vi "OFDM-A2信道估计.vi"(1 "信道2导频输入":cdb[](array[numeric])) -> (0 "输出":cdb[](array[numeric]))   [LabVIEW 2018]
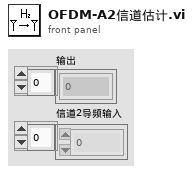
[diagram p1: front panel]
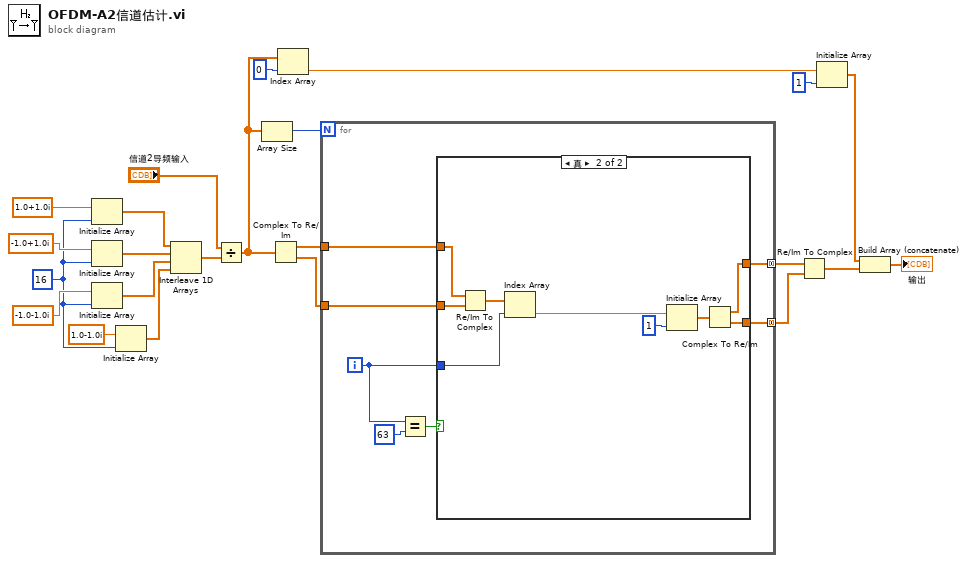
[diagram p0: block diagram]
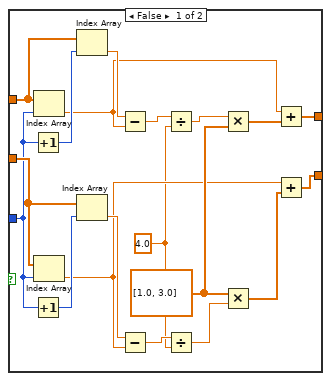
[diagram p2: hidden frame]
diagram:
  w2 = 16
  n1 = Initialize Array(cdb 1.0+1.0i, w2) -> (w9:cdb[])
  n2 = Initialize Array(cdb -1.0+1.0i, w2) -> (w6:cdb[])
  n3 = Initialize Array(cdb -1.0-1.0i, w2) -> (w7:cdb[])
  n4 = Initialize Array(cdb 1.0-1.0i, w2) -> (w8:cdb[])
  n5 = Interleave 1D Arrays(w9, w6, w7, w8) -> (w1:cdb[])
  n6 = Divide(x="信道2导频输入", y=w1) -> (x/y=w18:cdb[])
  n7 = Array Size(array=w18) -> (size(s)=w12:i32)
  n8 = Complex To Re/Im(x + iy=w18) -> (x=w23:dbl[], y=w22:dbl[])
  n9 = Index Array(array=w18, index=0) -> (element=w17:cdb)
  n10 = for {
    N: w12 -> [_]
    tunnel: w23 -> [w28]
    tunnel: w22 -> [w27]
    tunnel: [w24] -> w21 mode=concatenating
    tunnel: [w25] -> w20 mode=concatenating
    i -> [w26]
    n11 = Equal?(x=w26, y=63) -> (x = y?=w29:bool)
    n12 = case shown="真" w29 {
      tunnel: w28 -> [w49 w58]
      tunnel: w26 -> [w46 w55]
      tunnel: w27 -> [w47 w57]
      tunnel: [w33 w52] -> w24
      tunnel: [w32 w51] -> w25
      frame False {
        w31 = 4.0 ("y")
        w36 = dbl[] [1.0, 3.0] ("y")
        n13 = Increment(x=w46) -> (x+1=w48:i32)
        n14 = Increment(x=w46) -> (x+1=w45:i32)
        n15 = Index Array(array=w49, index=w46) -> (element=w40:dbl)
        n16 = Index Array(array=w47, index=w46) -> (element=w35:dbl)
        n17 = Index Array(array=w49, index=w48) -> (element=w44:dbl)
        n18 = Index Array(array=w47, index=w45) -> (element=w39:dbl)
        n19 = Subtract(x=w44, y=w40) -> (x-y=w43:dbl)
        n20 = Subtract(x=w39, y=w35) -> (x-y=w38:dbl)
        n21 = Divide(x=w43, y=w31) -> (x/y=w42:dbl)
        n22 = Divide(x=w38, y=w31) -> (x/y=w37:dbl)
        n23 = Multiply(x=w42, y=w36) -> (x*y=w41:dbl[])
        n24 = Multiply(x=w36, y=w37) -> (x*y=w34:dbl[])
        n25 = Add(x=w40, y=w41) -> (x+y=w33:dbl[])
        n26 = Add(x=w35, y=w34) -> (x+y=w32:dbl[])
      }
      frame True {
        n27 = Re/Im To Complex(1:w57, 2:w58) -> (0:w56:cdb[])
        n28 = Index Array(array=w56, index=w55) -> (element=w54:cdb)
        n29 = Initialize Array(w54, 1 ("维数大小")) -> (w53:cdb[])
        n30 = Complex To Re/Im(x + iy=w53) -> (x=w52:dbl[], y=w51:dbl[])
      }
    }
  }
  n31 = Re/Im To Complex(1:w20, 2:w21) -> (0:w13:cdb[])
  n32 = Initialize Array(w17, 1 ("维数大小")) -> (w14:cdb[])
  n33 = Build Array (concatenate)(w14, w13) -> (→"输出":cdb[])
